vi "Asana Dictionary Tasks Get Value.vi"(8 "error in (no error)":errorcluster, 10 "Key":string, 11 "data":T1(array[cluster])) -> (0 "error out":errorcluster, 3 "Value":string)   [LabVIEW 2019, in "Control Experiment.lvclass"]
uses:
  Control Experiment.lvclass
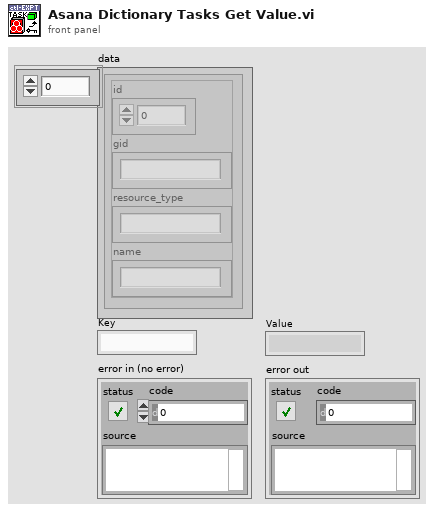
[diagram p1: front panel]
types:
  T1 = cluster{"id":i64, "gid":string, "resource_type":string, "name":string}[]
  T2 = typedef "Dictionary Object RefNum__ogtk.ctl" = refnum<k1>
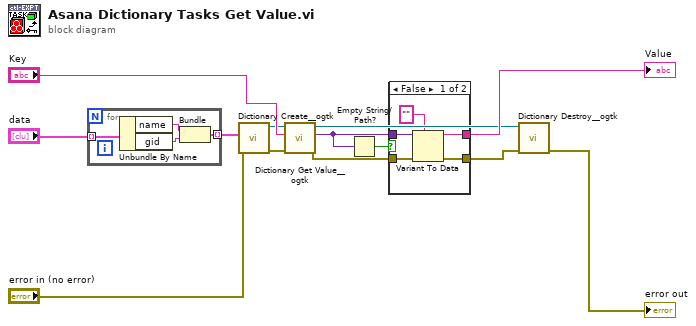
[diagram p0: block diagram]
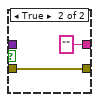
[diagram p2: hidden frame]
diagram:
  n1 = for {
    tunnel: "data" -> [w17] mode=indexing
    tunnel: [w14] -> w8 mode=indexing
    n2 = Unbundle By Name(w17) -> ("name"=w16:string, "gid"=w15:string)
    n3 = Bundle("name"=w16, "gid"=w15) -> (w14:cluster{"name":string, "gid":string})  [unwired: 1 in]
  }
  n4 = call <userlib>:"Dictionary Create__ogtk.vi"("error in (no error)"="error in (no error)", "initial dictionary (empty)"=w8) -> ("error out"=w5:errorcluster, "dictionary out"=w6:T2)  [unwired: 8 in]
  n5 = call <userlib>:"Dictionary Get Value__ogtk.vi"("error in"=w5, "key"="Key", "dictionary"=w6) -> ("error out"=w3:errorcluster, "value"=w2:variant, "dictionary out"=w11:T2)  [unwired: 5 in, 1 out]
  n6 = Empty String/Path?(string/path=w2) -> (empty?=w1:bool)
  n7 = case shown="False" w1 {
    tunnel: [w22 "" ("type")] -> w13
    tunnel: [w21 w24] -> w10
    tunnel: w3 -> [w20 w24]
    tunnel: w2 -> [w19 _]
    frame False {
      n8 = Variant To Data(error in=w20, type="", Variant=w19) -> (data=w22:string, error out=w21:errorcluster)
    }
    frame True {
    }
  }
  "Value" <- w13
  n9 = call <userlib>:"Dictionary Destroy__ogtk.vi"("error in (no error)"=w10, "dictionary"=w11) -> ("error out"=→"error out":errorcluster)  [unwired: 9 in]
